vi "43_Max_Area.vi"() -> ()   [LabVIEW 2018]
panel:
  in  "Stop":bool caption="Stop (F)"
  out "Image Out":T1(plugin-control)
  # "選出面積最大的"
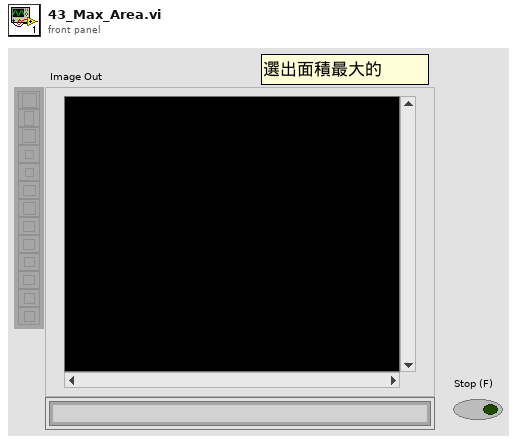
[diagram p1: front panel]
types:
  T1 = typedef "IMAQ Image.ctl" = refnum<image>
  T2 = cluster{"Left":dbl, "Top":dbl, "Right":dbl, "Bottom":dbl}
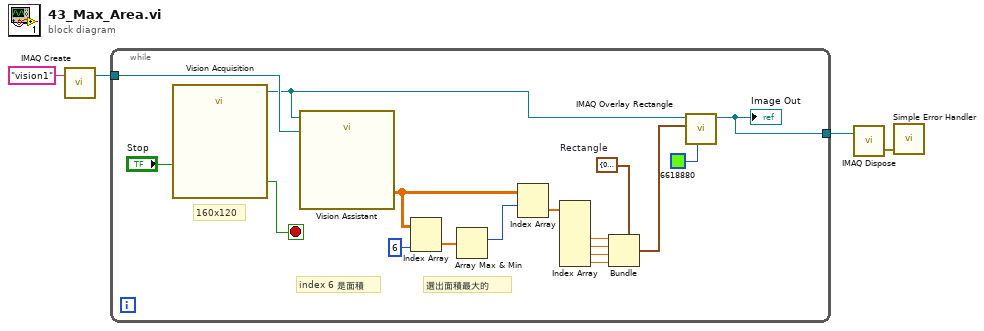
[diagram p0: block diagram]
diagram:
  n1 = call "IMAQ Create"("Image Name"="vision1") -> ("New Image"=w3:T1)  [unwired: 4 in, 1 out]
  n2 = while {
    tunnel: w3 -> [w11]
    tunnel: [w5] -> w1
    stop <- w20 stop-if-true
    w18 = T2 {"Left"=0.0, "Top"=0.0, "Right"=0.0, "Bottom"=0.0}  # Rectangle
    # "index 6 是面積"
    # "160x120"
    # "選出面積最大的"
    n3 = call "Vision Acquisition"("Stop (F)"="Stop") -> ("Image Out"=w10:T1, "Stopped"=w20:bool)  [unwired: 24 in, 1 out]
    n4 = call "Vision Assistant"("Image In"=w10, "Image Dst"=w11) -> ("Particle Measurements (Pixels) (Particle Analysis 1)"=w9:dbl[][])  [unwired: 22 in, 3 out]
    n5 = Index Array "Index Array"(array=w9, index (col)=6 ("disabled index (col)")) -> (element=w8:dbl[])  [unwired: 1 in]
    n6 = Array Max & Min(array=w8) -> (max index (indices)=w7:i32)  [unwired: 3 out]
    n7 = Index Array "Index Array"(array=w9, index (row)=w7) -> (element=w19:dbl[])  [unwired: 1 in]
    n8 = Index Array "Index Array"(array=w19) -> (element #3=w17:dbl, element #4=w16:dbl, element #5=w15:dbl, element #6=w14:dbl)  [unwired: 6 in, 2 out]
    n9 = Bundle "Bundle"(cluster=w18, "Left"=w17, "Top"=w16, "Right"=w15, "Bottom"=w14) -> (w13:T2)
    n10 = call "IMAQ Overlay Rectangle"("Color"=u32 6618880, "Rectangle"=w13, "Image"=w10) -> ("Image Out"=w5:T1)  [unwired: 7 in, 1 out]
    "Image Out" <- w5
  }
  n11 = call "IMAQ Dispose"("Image"=w1) -> ("error out"=w2:errorcluster)  [unwired: 5 in]
  n12 = call <vilib>:"Simple Error Handler.vi"("error in (no error)"=w2) -> ()  [unwired: 4 in, 5 out]
